vi "NumberArray.vi"   [LabVIEW 2009]
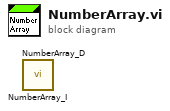
[diagram p0: block diagram]
diagram:
  n1 = call "NumberArray_I.vi"() -> ()  [unwired: 10 in, 2 out]
  n2 = call "NumberArray_D.vi"() -> ()  [unwired: 10 in, 2 out]
